vi "NI Car Monitor Narrow.vi"() -> ()   [LabVIEW 2018]
uses:
  <vilib>/Automotive Diagnostic Command Set/Diagnostic Transport.llb/Transport Protocol Selector.ctl
  <vilib>/xnet/xnet.llb/XNET Create Session (Frame Input Stream).vi
  <vilib>/addons/Automotive Diagnostic Command Set/NI_Automotive Diagnostic Command Set.lvlib
  <resource>/objmgr/xnet.rc
panel:
  in  "Start Monitor":bool
  in  "stop":bool
  in  "Tab Control":T1(tab)=enum."Interface Setup"
  out "车辆VIN码":string
  out "Mass Air Flow (g/s)":dbl(knob) scale=0.0..20000.0 scale format="%#_6p"
  out "Engine Load (%)":dbl(knob) scale=0.0..100.0
  out "Spark Advance (deg)":dbl(knob) scale=-90.0..90.0
  out "Air (degC)":dbl(slide) scale=0.0..150.0
  out "Throttle(%)":dbl(slide)=16.862745098039216 scale=0.0..100.0
  out "Engine (degC)":dbl(slide) scale=0.0..150.0
  out "Engine On Time (s)":u16
  in  "Update Rate (ms)":u32=50
  out "RPM":dbl(knob) scale=0.0..10000.0 scale format="%#_6p"
  out "Speed \n(km/hr)":dbl(knob) scale=0.0..250.0
  out "status":bool
  out "success?":bool
  out "MIL Lamp":u32 format="%.0x"
  out "Supported PIDs(2)":u8[](array[numeric])=[2, 3, 4, 5, 6, 7, 11, 12, 13] format="%x"
  out "永久的故障码":i32(listbox)
  out "Supported IDs(9)":u8[](array[numeric]) format="%x"
  out "当前激活的故障码":i32(listbox)
  out "激活的故障码":i32(listbox)
  out "Supported TIDs":u8[](array[numeric])=[1, 2, 32, 33, 64, 65, 66, 96, 128, 129] format="%x"
  out "Supported PIDs(1)":u8[](array[numeric])=[1, 3, 4, 5, 6, 7, 11, 12, 13, 14, 15, 17, 19, 20, 21, 28, 32, 33, 64, 71] format="%x"
  out "OBD Compliance Level":u16(ring) items=["(error)", "OBD II (California ARB)", "OBD (Federal EPA)", "OBD and OBD II", "OBD I", "Not OBD Compliant", "EOBD", "EBOD and OBD II", "EOBD and OBD", "EOBD, OBD, and OBDII", "JOBD", "JOBD and OBD II", "JOBD and EOBD", "JOBD, EOBD, and OBD II"]
  in  "Receive ID":u32=2024 format="%.0x"
  in  "Transmit ID":u32=2016 format="%.0x"
  in  "Baudrate":u32=500000
  in  "CAN Interface":string(combo)="CAN1"
  out "error out":errorcluster
  in  "HW select":u16(ring) items=["NI-XNET", "NI-CAN"]
  out "数组":T2(array[cluster])=[{"TID\n(测试方法)"=1, "TestValue"=3686, "Min limit"=3686, "Max limit"=3686, "DASID(转换)"=10}, {"TID\n(测试方法)"=1, "TestValue"=4928, "Min limit"=4928, "Max limit"=4928, "DASID(转换)"=10}, {"TID\n(测试方法)"=128, "TestValue"=1, "Min limit"=0, "Max limit"=0, "DASID(转换)"=0}, {"TID\n(测试方法)"=129, "TestValue"=0, "Min limit"=0, "Max limit"=22272, "DASID(转换)"=5}, {"TID\n(测试方法)"=192, "TestValue"=1, "Min limit"=0, "Max limit"=0, "DASID(转换)"=0}, {"TID\n(测试方法)"=161, "TestValue"=132, "Min limit"=0, "Max limit"=9108, "DASID(转换)"=20}, {"TID\n(测试方法)"=161, "TestValue"=90, "Min limit"=0, "Max limit"=1218, "DASID(转换)"=20}, {"TID\n(测试方法)"=0, "TestValue"=1, "Min limit"=0, "Max limit"=0, "DASID(转换)"=0}, {"TID\n(测试方法)"=128, "TestValue"=0, "Min limit"=0, "Max limit"=0, "DASID(转换)"=0}, {"TID\n(测试方法)"=130, "TestValue"=32927, "Min limit"=25231, "Max limit"=40305, "DASID(转换)"=5}] {"TID\n(测试方法)" format="%.0x"; "DASID(转换)" format="%.0x"}
  # "排放监控1"
  # "排放监控2"
  # "催化剂监控1"
  # "排放加热监控1"
  # "排放加热监控2"
  # "燃料系统监控1"
  # "从稀到浓传感器阈值电压"
  # "厂家定义"
  # "厂家定义"
  # "厂家定义"
  # "厂家定义"
  # "*0.1220703125(mV)"
  # "*1(ohm)"
  # "*0.000030517578"
  # "*0.000030517578(signed)"
  # "The NI OBD-II Car Monitor is for demonstration purposes only. No guarantee  is made to the accuracy or compatibilty of this example, and\nno support is offered for this demo.\n\nHardware: \nThis application works with NI-XNET and NI-CAN HW. NI USB, cDAQ, cRIO, PXI, PCI, and PCMCIA CAN interfaces. \n\nTo build a custom application like this, you need LabVIEW 2009 or later, the Automotive Diagnostic Command Set, and an NI-CAN or NI-XNET interface.\nYou can find all of these products at http://ni.com/CAN\n\nTo Begin: Configure your interface in the Interface Setup tab, Click Start Monitor, and go to the Real Time Display Tab."
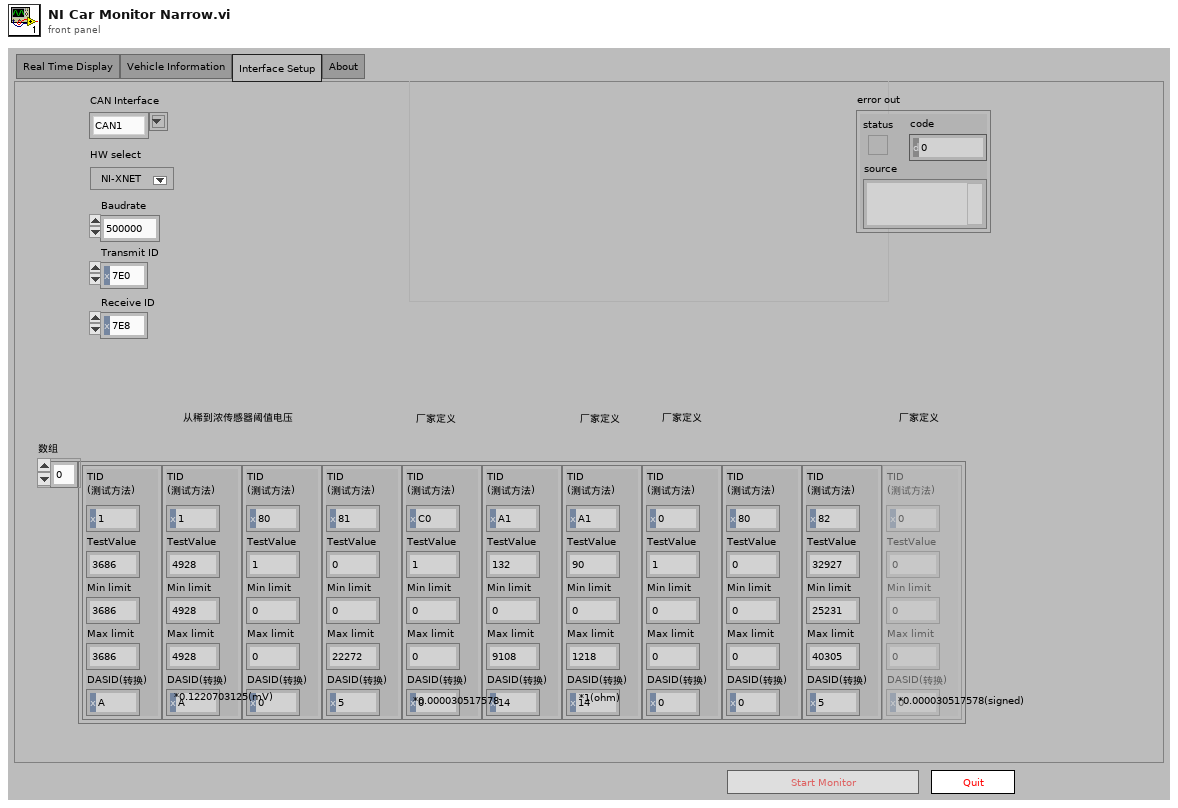
[diagram p1: front panel]
types:
  T1 = enum32{"Real Time Display", "Vehicle Information", "Interface Setup", "About"}
  T2 = cluster{"TID\n(测试方法)":u8, "TestValue":u16, "Min limit":u16, "Max limit":u16, "DASID(转换)":u8}[]
  T3 = typedef "NI_Automotive Diagnostic Command Set.lvlib/Transport Protocol Selector.ctl" = enum16{"ISO TP - Normal Mode", "ISO TP - Mixed Mode", "VW TP 2.0", "Diagnostics on IP", "ISO TP LIN"}
  T4 = typedef "NI_Automotive Diagnostic Command Set.lvlib/Diag Reference.ctl" = cluster{"Diag CAN Handle":u32, "Transport Protocol":T3, "Receive Address Extension":u8, "Transmit Address Extension":u8, "Receive CAN Id":u32, "Transmit CAN Id":u32, "Log Frames ?":bool, "My TP Address":u8, "Other TP Address":u8, "T1":u16, "T2":u16, "T3":u16, "T4":u16, "Tx SN":u8, "Block Size":u8, "Rx SN":u8, "VW TP Initialized?":bool, "Tx block no":u8, "baud rate":u64, "Interface":string, "Channel Diag CAN Handle":u32, "UDP Connection ID":refnum<k16>, "TCP Connection ID":refnum<k5>, "Target IP Addr":u32, "Source Address":u16, "Target Address":u16, "Send Header NACK?":bool, "DLL Handle":u32, "NAD":u8, "Time Stamp read first":dbl, "Time Stamp read last":dbl, "Time Stamp write first":dbl, "Time Stamp write last":dbl, "Time Stamp write":dbl, "Time Stamp read":dbl, " I/O Mode":u32, "FD Baudrate":u64, "TX_DL":u16, "RX_DL":u16, "DoIP Protocol Version":T5, " Selected I/O Mode":u32, "TesterPresent Counter":u32, "TesterPresent Limit":u32, "TesterPresent Tick[ms]":i32, "TesterPresent RequireResponse?":bool, "TesterPresent Stored Ref?":bool, "TesterPresent Message":u8[], "TesterPresent Task Handle":i32, "TesterPresent Semaphore":T6, "Response Plausibility Check":u32, "Default Version?":bool, "Diagostic Globals":T7, "Session-based Properties?":bool}
  T5 = typedef "NI_Automotive Diagnostic Command Set.lvlib/DoIP Protocol Version.ctl" = u8
  T6 = typedef "Semaphore RefNum" = refnum<k1>
  T7 = typedef "NI_Automotive Diagnostic Command Set.lvlib/Diag Globals.ctl" = cluster{"Timeout FC (Bs)":u32, "Timeout CF (Cr)":u32, "Timeout Diag Command":u32, "Receive Block Size (BS)":u8, "Wait Time CF (STmin)":u8, "Max Waits (N_WFTmax)":u8, "Waits to Send (N_WAIT)":i32, "Time between Waits (TW)":u32, "Fill CAN Frames?":bool, "Fill Byte":u32, "Invalid Response as Error?":bool, "Max RspPending Count":u32, "VWTP Command Timeout":u32, "Transport Protocol":T3, "Diag CAN Handle":u32, "DLL Handle":u32, "Timeout RspPending":u32}
  T8 = typedef "OBD Data Typedef.ctl" = cluster{"Engine RPM":dbl, "Time Since Engine Start (s)":dbl, "km/hr":dbl, "Engine Load (%)":dbl, "Engine Coolant Temp(ºC)":dbl, "Intake Air Temp (DegC)":dbl, "MAF Rate (g/s)":dbl, "Throttle Position (%)":dbl, "Timing Advance (º)":dbl, "MIL Lamp":u32, "OBD Compliance Level":u16}
  T9 = cluster{"TID":u8, "组件ID":u8, "LimitType":enum16{"MaxLimit", "MinLimit"}, "TestValue":u16, "Limit":u16}
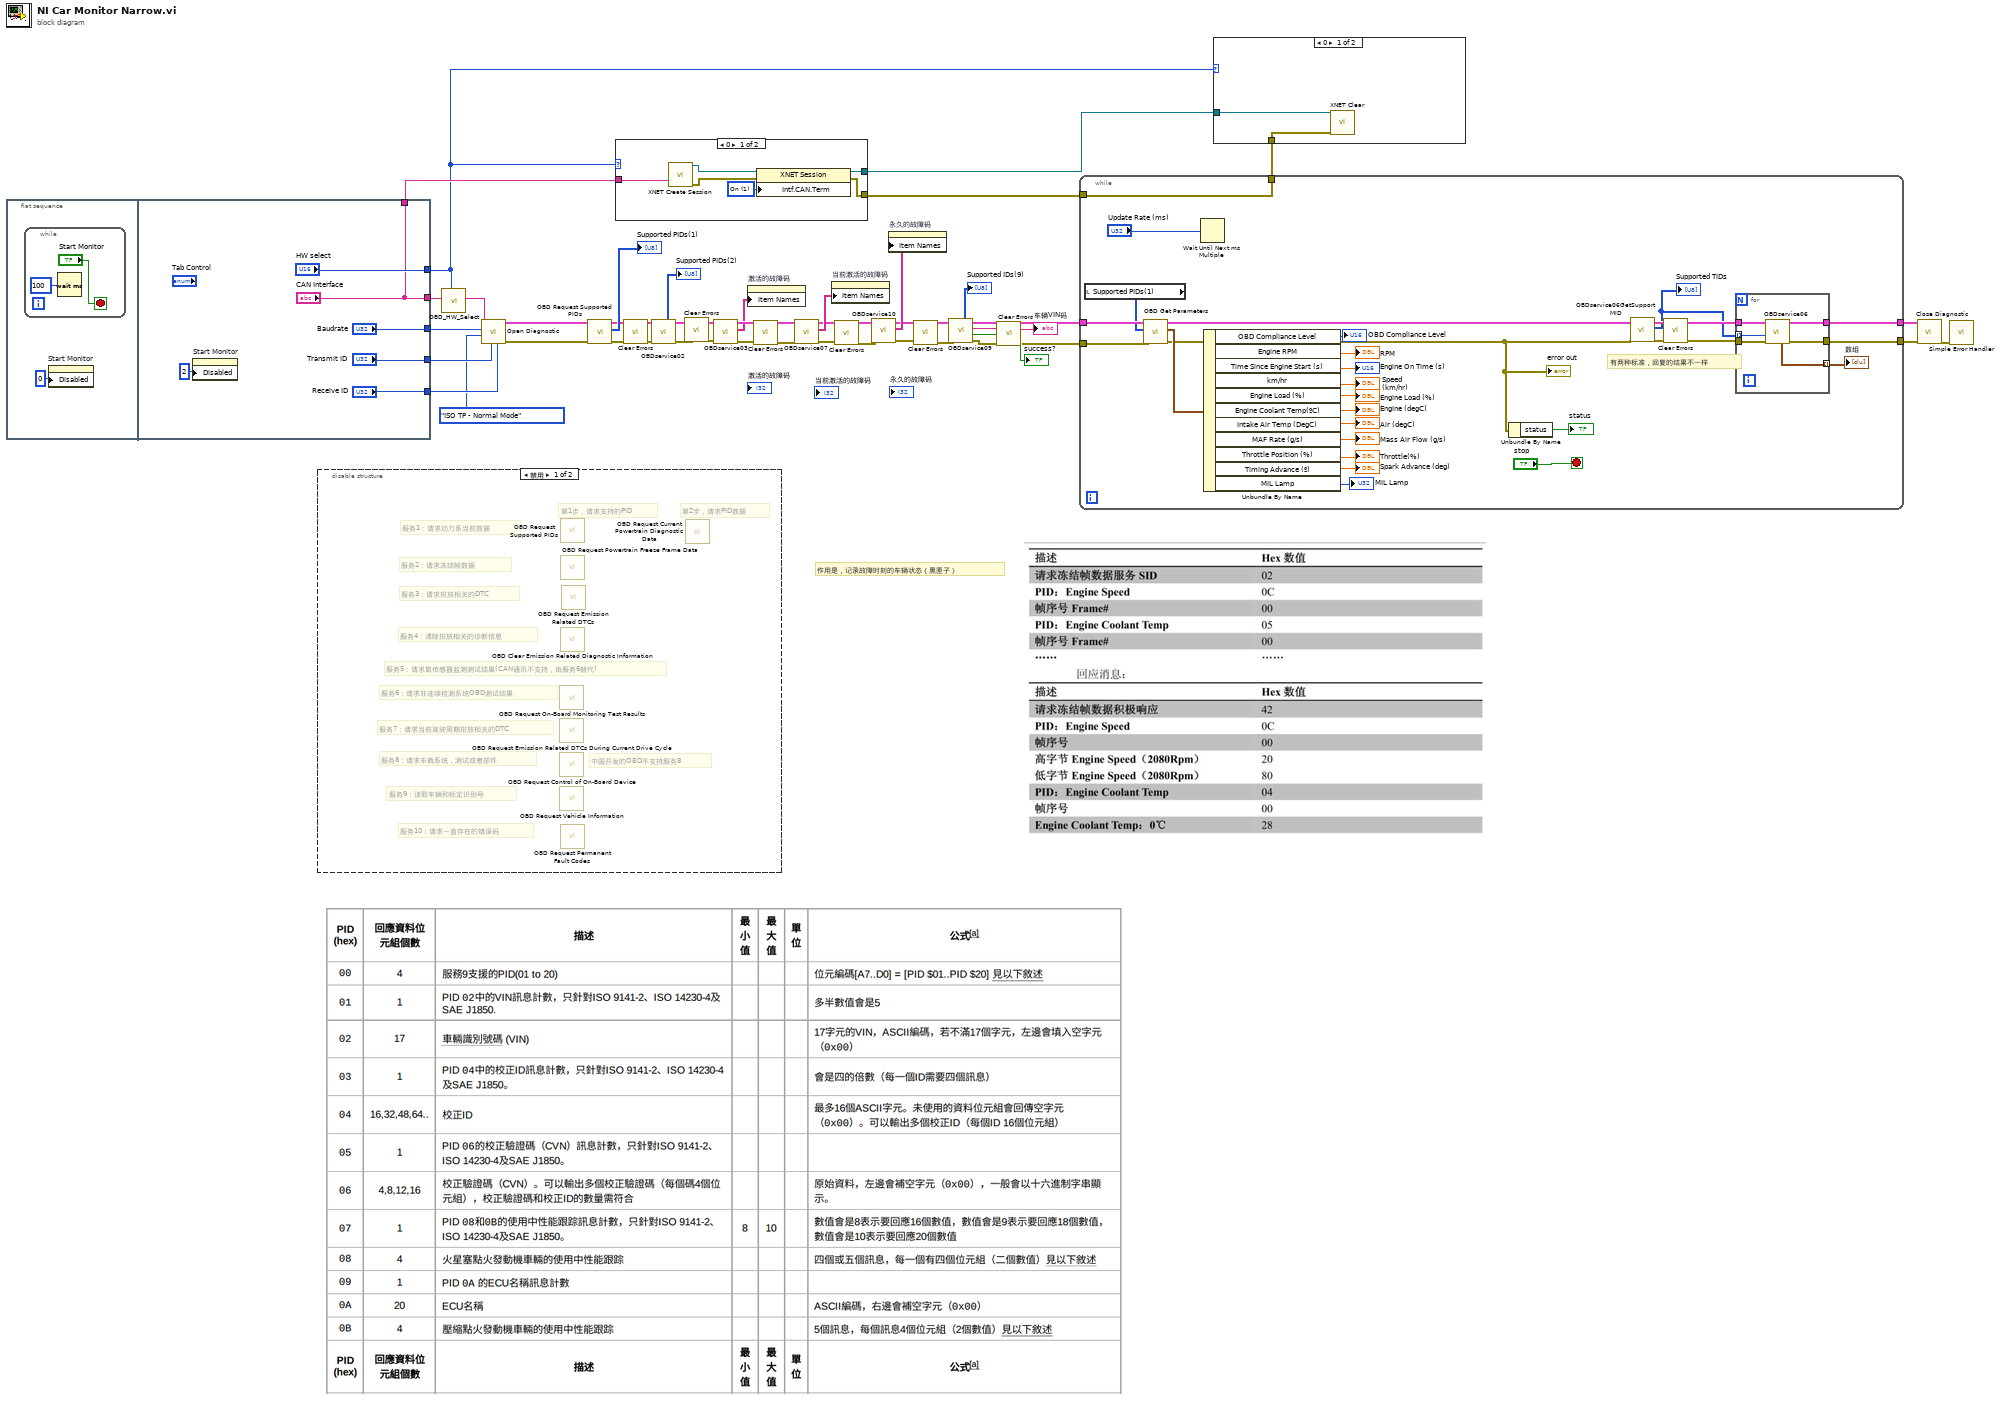
[diagram p0: block diagram]
diagram:
  # "作用是，记录故障时刻的车辆状态（黑匣子）"
  n1 = flat-sequence {
    tunnel: ["Receive ID"] -> w37
    tunnel: ["Transmit ID"] -> w36
    tunnel: ["Baudrate"] -> w35
    tunnel: ["CAN Interface"] -> w34
    tunnel: ["HW select"] -> w30
    tunnel: ["CAN Interface"] -> w31
    frame #0 {
      n2 = while {
        stop <- "Start Monitor" stop-if-true
        n3 = Wait (ms)(milliseconds to wait=u32 100) -> ()  [unwired: 1 out]
      }
      n4 = property on="Start Monitor" class="Bool"("Disabled"=u8 0) -> ()  [unwired: 2 in, 2 out]
    }
    frame #1 {
      n5 = property on="Start Monitor" class="Bool"("Disabled"=u8 2) -> ()  [unwired: 2 in, 2 out]
    }
  }
  n6 = disable-structure shown="禁用" {
    frame Disabled {
      # "中国开发的OBD不支持服务8"
      # "服务5：请求氧传感器监测测试结果(CAN通讯不支持，由服务6替代)"
      # "服务8：请求车载系统，测试或者部件"
      # "服务9：读取车辆和标定识别号"
      # "服务10：请求一直存在的错误码"
      # "服务7：请求当前驾驶周期排放相关的DTC"
      # "服务6：请求非连续检测系统OBD测试结果"
      # "服务4：清除排放相关的诊断信息"
      # "服务3：请求排放相关的DTC"
      # "服务2：请求冻结帧数据"
      # "第2步，请求PID数据"
      # "第1步，请求支持的PID"
      # "服务1：请求动力系当前数据"
      n7 = call <vilib>:"OBD Request On-Board Monitoring Test Results.vi"() -> ()  [unwired: 8 in, 4 out]
      n8 = call <vilib>:"OBD Request Emission Related DTCs During Current Drive Cycle.vi"() -> ()  [unwired: 8 in, 4 out]
      n9 = call <vilib>:"OBD Request Control of On-Board Device.vi"() -> ()  [unwired: 8 in, 4 out]
      n10 = call <vilib>:"OBD Request Vehicle Information.vi"() -> ()  [unwired: 7 in, 5 out]
      n11 = call <vilib>:"OBD Request Supported PIDs.vi"() -> ()  [unwired: 9 in, 3 out]
      n12 = call <vilib>:"OBD Request Powertrain Freeze Frame Data.vi"() -> ()  [unwired: 8 in, 4 out]
      n13 = call <vilib>:"OBD Clear Emission Related Diagnostic Information.vi"() -> ()  [unwired: 9 in, 3 out]
      n14 = call <vilib>:"OBD Request Permanent Fault Codes.vi"() -> ()  [unwired: 8 in, 4 out]
      n15 = call <vilib>:"OBD Request Emission Related DTCs.vi"() -> ()  [unwired: 8 in, 4 out]
      n16 = call <vilib>:"OBD Request Current Powertrain Diagnostic Data.vi"() -> ()  [unwired: 8 in, 4 out]
    }
    frame Enabled {
    }
  }
  n17 = call "OBD_HW_Select.vi"("HW select"=w30, "CAN port"=w34) -> ("CAN port out"=w39:string)  [unwired: 9 in]
  n18 = call <vilib>:"Open Diagnostic.vi"("Receive ID"=w37, "Transmit ID"=w36, "Transport Protocol"=Transport_Protocol_Selector."ISO TP - Normal Mode", "Baud Rate"=w35, "CAN Interface"=w39) -> ("error out"=w1:errorcluster, "diag ref out"=w2:T4)  [unwired: 5 in]
  n19 = call <vilib>:"OBD Request Supported PIDs.vi"("error in (no error)"=w1, "diag ref in"=w2) -> ("error out"=w11:errorcluster, "PIDs out"=→"Supported PIDs(1)":u8[], "diag ref out"=w18:T4)  [unwired: 7 in]
  n20 = case shown="0" w30 {
    tunnel: w31 -> [w57 _]
    tunnel: [w53 _] -> w27
    tunnel: [w52 _] -> w28
    frame 0 {
      w54 = u32 1 items=["Off", "On"] ("Interface:CAN:Termination")
      n21 = call-poly <vilib>:"XNET Create Session.vi"("interface"=w57) -> ("session out"=w56:refnum<k21>, "error out"=w55:errorcluster)  [unwired: 13 in]
      n22 = property class="XNET Session"(reference=w56, error in=w55, "Intf.CAN.Term"=w54) -> (reference out=w53:refnum<k21>, error out=w52:errorcluster)
    }
    frame 1, Default {
    }
  }
  n23 = call <vilib>:"Clear Errors.vi"("error in (no error)"=w11) -> ("error out"=w10:errorcluster)  [unwired: 5 in, 1 out]
  n24 = call "OBDservice02.vi"("错误输入（无错误）"=w10, "diag ref out输入"=w18) -> ("错误输出"=w9:errorcluster, "diag ref out输出"=w17:T4, "PIDs out"=→"Supported PIDs(2)":u8[])  [unwired: 5 in, 2 out]
  n25 = call <vilib>:"Clear Errors.vi"("error in (no error)"=w9) -> ("error out"=w8:errorcluster)  [unwired: 5 in, 1 out]
  n26 = call "OBDservice03.vi"("错误输入（无错误）"=w8, "diag ref out输入"=w17) -> ("错误输出"=w7:errorcluster, "dtcs"=w23:string[], "diag ref out输出"=w24:T4)  [unwired: 6 in, 1 out]
  n27 = property on="激活的故障码" class="LstBox (严格)"("Item Names"=w23) -> ()  [unwired: 2 in, 2 out]
  n28 = call <vilib>:"Clear Errors.vi"("error in (no error)"=w7) -> ("error out"=w6:errorcluster)  [unwired: 5 in, 1 out]
  n29 = call "OBDservice07.vi"("错误输入（无错误）"=w6, "diag ref out输入"=w24) -> ("错误输出"=w5:errorcluster, "dtcs"=w22:string[], "diag ref out"=w21:T4)  [unwired: 6 in, 1 out]
  n30 = property on="当前激活的故障码" class="LstBox (严格)"("Item Names"=w22) -> ()  [unwired: 2 in, 2 out]
  n31 = call <vilib>:"Clear Errors.vi"("error in (no error)"=w5) -> ("error out"=w12:errorcluster)  [unwired: 5 in, 1 out]
  n32 = call "OBDservice10.vi"("错误输入（无错误）"=w12, "diag ref out输入"=w21) -> ("错误输出"=w14:errorcluster, "dtcs"=w20:string[], "diag ref out"=w19:T4)  [unwired: 6 in, 1 out]
  n33 = property on="永久的故障码" class="LstBox (严格)"("Item Names"=w20) -> ()  [unwired: 2 in, 2 out]
  n34 = call <vilib>:"Clear Errors.vi"("error in (no error)"=w14) -> ("error out"=w13:errorcluster)  [unwired: 5 in, 1 out]
  n35 = call "OBDservice09.vi"("错误输入（无错误）"=w13, "diag ref out输入"=w19) -> ("错误输出"=w4:errorcluster, "success?"=→"success?":bool, "string"=→"车辆VIN码":string, "diag ref out输出"=w32:T4, "MIDs out"=→"Supported IDs(9)":u8[])  [unwired: 5 in]
  n36 = call <vilib>:"Clear Errors.vi"("error in (no error)"=w4) -> ("error out"=w3:errorcluster)  [unwired: 5 in, 1 out]
  n37 = while {
    tunnel: w32 -> [w82]
    tunnel: [w69] -> w42
    tunnel: [w70] -> w41
    tunnel: [w72] -> w29
    tunnel: w28 -> [w72]
    tunnel: w3 -> [w64]
    stop <- "stop" stop-if-true
    # "有两种标准，回复的结果不一样"
    n38 = local read "Supported PIDs(1)"() -> (w66:u8[])
    n39 = call "OBD Get Parameters.vi"("Error In"=w64, "Supported PIDs"=w66, "diag ref in"=w82) -> ("error out"=w59:errorcluster, "Diagnostic Data"=w68:T8, "diag ref out"=w62:T4)  [unwired: 5 in]
    "error out" <- w59
    n40 = Wait Until Next ms Multiple(millisecond multiple="Update Rate (ms)") -> ()  [unwired: 1 out]
    n41 = Unbundle By Name(w68) -> ("OBD Compliance Level"=→"OBD Compliance Level":u16, "Engine RPM"=→"RPM":dbl, "Time Since Engine Start (s)"=→"Engine On Time (s)":dbl, "km/hr"=→"Speed \n(km/hr)":dbl, "Engine Load (%)"=→"Engine Load (%)":dbl, "Engine Coolant Temp(ºC)"=→"Engine (degC)":dbl, "Intake Air Temp (DegC)"=→"Air (degC)":dbl, "MAF Rate (g/s)"=→"Mass Air Flow (g/s)":dbl, "Throttle Position (%)"=→"Throttle(%)":dbl, "Timing Advance (º)"=→"Spark Advance (deg)":dbl, "MIL Lamp"=→"MIL Lamp":u32)
    n42 = Unbundle By Name(w59) -> ("status"=→"status":bool)
    n43 = call "OBDservice06GetSupportMID.vi"("error in (no error) 2"=w59, "diag ref in"=w62) -> ("error out 2"=w63:errorcluster, "MIDs out"=w60:u8[], "diag ref out 2"=w61:T4)  [unwired: 6 in, 1 out]
    "Supported TIDs" <- w60
    n44 = call <vilib>:"Clear Errors.vi"("error in (no error)"=w63) -> ("error out"=w58:errorcluster)  [unwired: 5 in, 1 out]
    n45 = for {
      tunnel: w61 -> [w91]
      tunnel: w60 -> [w90] mode=indexing
      tunnel: w58 -> [w89]
      tunnel: [w88] -> w69
      tunnel: [w87] -> w70
      tunnel: [w86] -> w71 mode=indexing
      n46 = call "OBDservice06.vi"("error in (no error)"=w89, "data"=w90, "diag ref in 2"=w91) -> ("error out"=w87:errorcluster, "diag ref out"=w88:T4, "data"=w86:T9)  [unwired: 4 in, 2 out]
    }
    "数组" <- w71
  }
  n47 = case shown="0" w30 {
    tunnel: w29 -> [w93 _]
    tunnel: w27 -> [w92 _]
    frame 0 {
      n48 = call <vilib>:"XNET Clear.vi"("session in"=w92, "error in (no error)"=w93) -> ()  [unwired: 13 in, 1 out]
    }
    frame 1, Default {
    }
  }
  n49 = call <vilib>:"Close Diagnostic.vi"("error in (no error)"=w41, "diag ref in"=w42) -> ("error out"=w40:errorcluster)  [unwired: 9 in]
  n50 = call <vilib>:"Simple Error Handler.vi"("error in (no error)"=w40) -> ()  [unwired: 4 in, 5 out]
